vi "disconnect.vi"(8 "error in":errorcluster, 9 "timeout (5000)":i32=5000, 11 "websocket client in":refnum<class "websocket client.lvclass">) -> (0 "error out":errorcluster, 2 "final messages":string[](array[string]), 3 "websocket client out":refnum<class "websocket client.lvclass">)   [LabVIEW 2016, in "websocket client.lvclass"]
uses:
  websocket client.lvclass
  websocket core.lvlib
  lvlibtls/socket connection/lvlibretls connection.lvclass
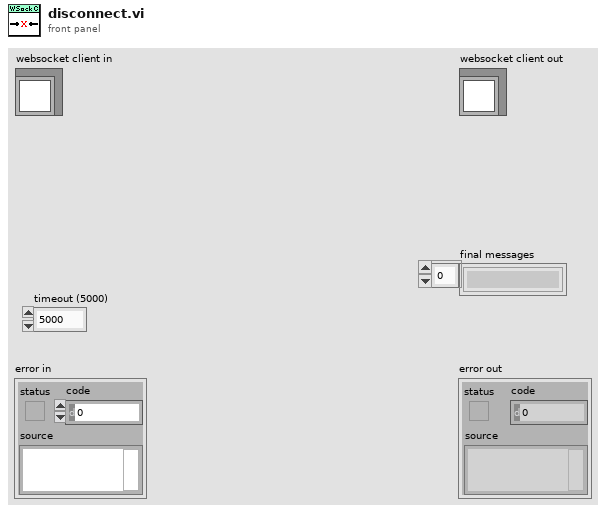
[diagram p1: front panel]
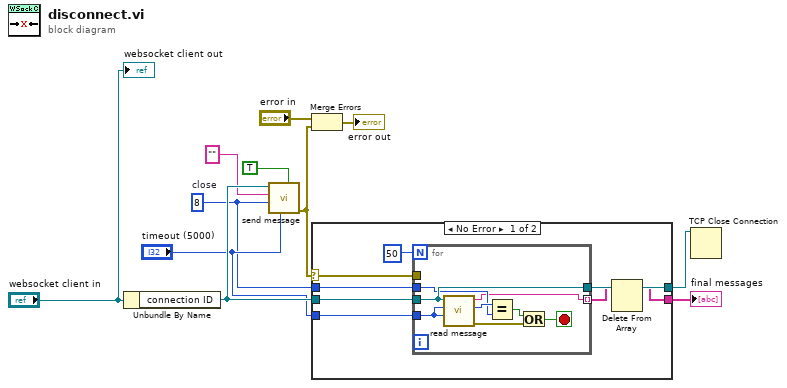
[diagram p0: block diagram]
diagram:
  w2 = u8 8  # close
  n1 = Unbundle By Name("websocket client in") -> ("connection ID"=w9:refnum<k5>)
  n2 = call "send message.vi"("mask? (F)"=TRUE, "timeout ms (5000)"="timeout (5000)", "opcode"=w2, "data"="", "lvlibretls connection in"=w9) -> ("error out"=w4:errorcluster)  [unwired: 5 in, 1 out]
  n3 = Merge Errors("error in", w4) -> (→"error out":errorcluster)
  n4 = case shown="No Error" w4 {
    selector: w4 -> [w17 _]
    tunnel: w9 -> [w19 w28]
    tunnel: [w18 w28] -> w6
    tunnel: "timeout (5000)" -> [w16 _]
    tunnel: w2 -> [w15 _]
    tunnel: [w13 _] -> w1
    frame No Error {
      n5 = for {
        N: 50 -> [_]
        tunnel: w19 -> [w26]
        tunnel: w17 -> [_]
        tunnel: [w26] -> w18
        tunnel: w16 -> [w25]
        tunnel: w15 -> [w23]
        tunnel: [w20] -> w12 mode=indexing
        stop <- w21 stop-if-true
        n6 = call "read message.vi"("continuation timeout (10000)"=w25, "base timeout (5000)"=w25, "tcp connection"=w26) -> ("error"=w27:errorcluster, "Numeric"=w24:u8, "message"=w20:string)  [unwired: 6 in]
        n7 = Equal?(x=w24, y=w23) -> (x = y?=w22:bool)
        n8 = Or(x=w22, y=w27) -> (x .or. y?=w21:bool)
      }
      n9 = Delete From Array(array=w12) -> (array with subset deleted=w13:string[])  [unwired: 2 in, 1 out]
    }
    frame Error {
    }
  }
  "final messages" <- w1
  n10 = TCP Close Connection(connection ID=w6) -> ()  [unwired: 2 in, 2 out]
  "websocket client out" <- "websocket client in"
